vi "Include Path Xcontrol.vi"() -> ()   [LabVIEW 2013]
uses:
  <resource>/importtools/Common/Include Paths Control/NISAST Include Paths.xctl
panel:
  in  "NISAST包括路径":string[](xcontrol)
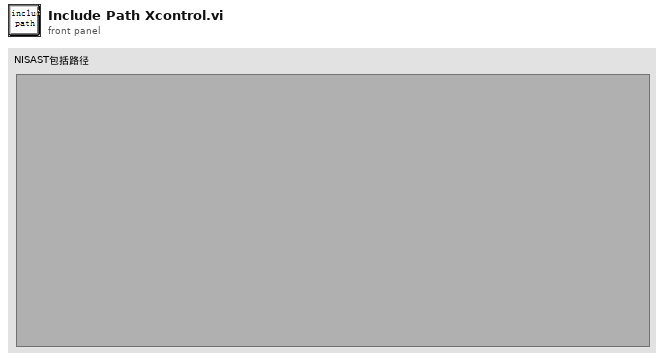
[diagram p1: front panel]
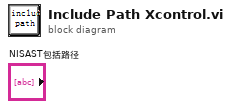
[diagram p0: block diagram]
diagram:
